vi "calculate deltaXbead of tether .vi"() -> ()   [LabVIEW 2014]
uses:
  <vilib>/Utility/file.llb/Read From Spreadsheet File (DBL).vi
  <vilib>/Utility/file.llb/Write To Spreadsheet File (DBL).vi
panel:
  in  "save?":bool
  in  "Tab Control":enum32{"Page 1", "Page 2"}(tab)
  out "bead position vs deltaXbead":T1(graph)
  in  "X=T; Y=F":bool
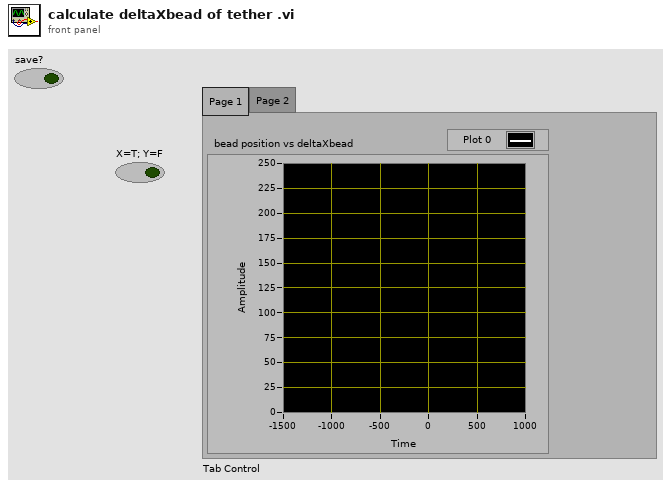
[diagram p1: front panel]
types:
  T1 = cluster{"bead position (nm)":dbl[], "delta Xbead":dbl[]}
  T2 = typedef "(1+2+3)fit stuckbead coefficient.ctl" = cluster{"(1)stuckbead-scan coefficient ":dbl[], "(2)stuckbead-scan coefficient ":dbl[], "(3)stuckbead-scan coefficient":dbl[]}
  T3 = cluster{"bead position out (nm)":dbl[], "delta Xbead (nm)":dbl[]}
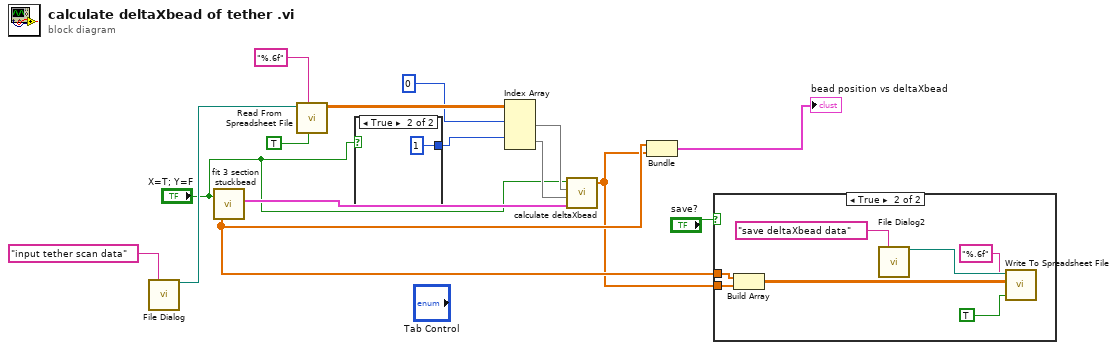
[diagram p0: block diagram]
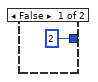
[diagram p3: hidden frame]
diagram:
  n1 = call "File Dialog"("prompt"="input tether scan data") -> ("selected path"=w13:path)  [unwired: 11 in, 3 out]
  n2 = call "fit 3 section stuckbead.vi"("X=T; Y=F"="X=T; Y=F") -> ("bead position out (nm)"=w3:dbl[], "(1+2+3) stuckbead-scan coefficient"=w15:T2)  [unwired: 3 out]
  n3 = call-poly <vilib>:"Read From Spreadsheet File.vi"("transpose (no:F)"=TRUE, "format (%.3f)"="%.6f", "file path (dialog if empty)"=w13) -> ("all rows"=w12:dbl[][])  [unwired: 4 in, 4 out]
  n4 = case shown="True" "X=T; Y=F" {
    tunnel: [2 1] -> w9
    frame False {
    }
    frame True {
    }
  }
  n5 = Index Array(array=w12, index (row) #1=0 ("index (row)"), index (row) #2=w9) -> (element #1=w8:dbl[], element #2=w7:dbl[])  [unwired: 2 in]
  n6 = call "calculate deltaXbead.vi"("X=T; Y=F"="X=T; Y=F", "Stage position (um)"=w8, "QPD signal (V)"=w7, "(1+2+3) stuckbead-scan coefficient"=w15) -> ("delta Xbead (nm)"=w2:dbl[])  [unwired: 2 in, 1 out]
  n7 = Bundle("bead position out (nm)"=w3, "delta Xbead (nm)"=w2) -> (→"bead position vs deltaXbead":T3)  [unwired: 1 in]
  n8 = case shown="True" "save?" {
    tunnel: w3 -> [_ w22]
    tunnel: w2 -> [_ w21]
    frame False {
    }
    frame True {
      n9 = Build Array(w22, w21) -> (w24:dbl[][])
      n10 = call "File Dialog2"("prompt"="save deltaXbead data") -> ("selected path"=w19:path)  [unwired: 11 in, 3 out]
      n11 = call-poly <vilib>:"Write To Spreadsheet File.vi"("transpose? (no:F)"=TRUE, "format (%.3f)"="%.6f", "2D data"=w24, "file path (dialog if empty)"=w19) -> ()  [unwired: 4 in, 1 out]
    }
  }
